vi "Base Error Code.vi"() -> (3 "base error code":i32)   [LabVIEW 2021, in "DSF Core.lvlib" / "Framework.lvclass"]
uses:
  Classes/Framework/Framework.lvclass
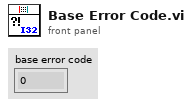
[diagram p1: front panel]
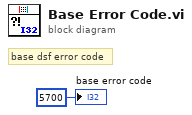
[diagram p0: block diagram]
diagram:
  # "base dsf error code"
  "base error code" <- 5700 ("base error code")
